vi "calc_floc_sat.vi"(11 "RowData":T1) -> (3 "RowData 2":T1)   [LabVIEW 2019]
uses:
  RowData_Type.ctl
  Global Plantita Parameters.vi
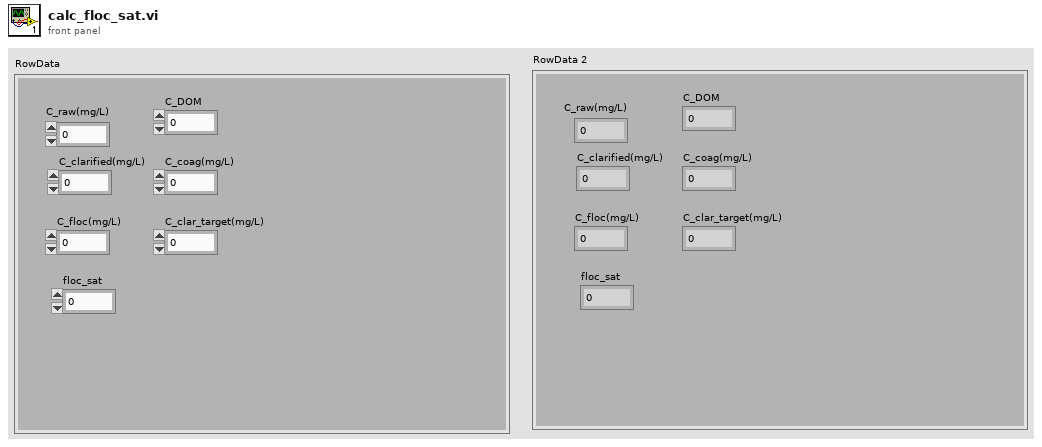
[diagram p1: front panel]
types:
  T1 = typedef "RowData_Type.ctl" = cluster{"C_raw(mg/L)":dbl, "C_clarified(mg/L)":dbl, "C_floc(mg/L)":dbl, "floc_sat":dbl, "C_DOM":dbl, "C_coag(mg/L)":dbl, "C_clar_target(mg/L)":dbl}
  T2 = cluster{"height_ff (m)":dbl, "C_coag_stock (g/L)":dbl, "flocculation_time(min)":dbl, "clarification_time(min)":dbl, "data_interval (min)":dbl, "kpf":dbl, "kc":dbl, "q":dbl}
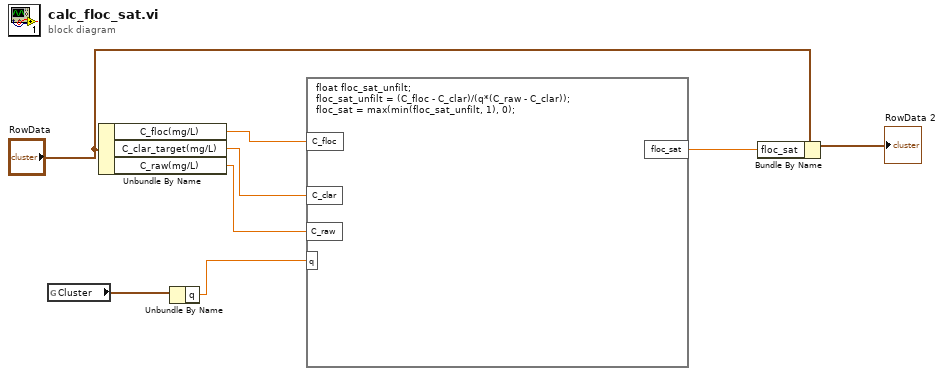
[diagram p0: block diagram]
diagram:
  n1 = global read "Global Plantita Parameters.vi" "Cluster"() -> (w2:T2)
  n2 = Unbundle By Name("RowData") -> ("C_floc(mg/L)"=w8:dbl, "C_clar_target(mg/L)"=w7:dbl, "C_raw(mg/L)"=w3:dbl)
  n3 = Unbundle By Name(w2) -> ("q"=w1:dbl)
  n4 = formula code="float floc_sat_unfilt;\nfloc_sat_unfilt = (C_floc - C_clar)/(q*(C_raw - C_clar));\nfloc_sat = max(min(floc_sat_unfilt, 1), 0);"("C_floc"=w8, "C_clar"=w7, "q"=w1, "C_raw"=w3) -> ("floc_sat"=w4:dbl)
  n5 = Bundle By Name(cluster="RowData", "floc_sat"=w4) -> (→"RowData 2":T1)
